vi "Convert-U8-for-Logging.vi"(11 "u8 Array":u8[](array[numeric]) format="%.0x") -> (3 "Output String":string)   [LabVIEW 2018]
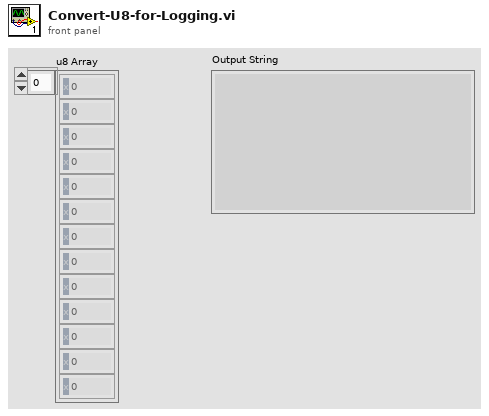
[diagram p1: front panel]
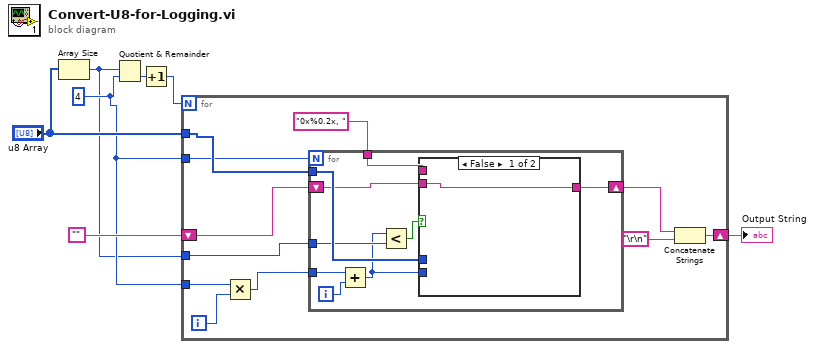
[diagram p0: block diagram]
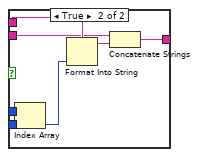
[diagram p2: hidden frame]
diagram:
  w2 = 4 ("y")
  n1 = Array Size(array="u8 Array") -> (size(s)=w1:i32)
  n2 = Quotient & Remainder(x=w1, y=w2) -> (floor(x/y)=w4:i32)  [unwired: 1 out]
  n3 = Increment(x=w4) -> (x+1=w3:i32)
  n4 = for {
    N: w3 -> [_]
    shift-right: [w10] -> w6
    shift-left: "" -> [w13]
    tunnel: "u8 Array" -> [w14]
    tunnel: w2 -> [w17]
    tunnel: w2 -> [w12]
    tunnel: w1 -> [w8]
    i -> [w18]
    n5 = Multiply(x=w17, y=w18) -> (x*y=w16:i32)
    n6 = for {
      N: w12 -> [_]
      tunnel: w16 -> [w26]
      tunnel: "0x%0.2x, " ("format string") -> [w25]
      tunnel: w14 -> [w24]
      shift-right: [w22] -> w11
      shift-left: w13 -> [w23]
      tunnel: w8 -> [w21]
      i -> [w27]
      n7 = Add(x=w26, y=w27) -> (x+y=w20:i32)
      n8 = Less?(x=w20, y=w21) -> (x < y?=w19:bool)
      n9 = case shown="False" w19 {
        tunnel: w25 -> [_ w35]
        tunnel: w24 -> [_ w34]
        tunnel: w23 -> [w28 w32]
        tunnel: [w28 w30] -> w22
        tunnel: w20 -> [_ w29]
        frame False {
        }
        frame True {
          n10 = Index Array(array=w34, index=w29) -> (element=w33:u8)
          n11 = Format Into String(format string=w35, w33) -> (resulting string=w31:string)  [unwired: 2 in, 1 out]
          n12 = Concatenate Strings(w32, w31) -> (w30:string)
        }
      }
    }
    n13 = Concatenate Strings(w11, "\r\n") -> (w10:string)
  }
  "Output String" <- w6
